vi "AOTF-Trigger_1.vi"(0 "Channel":string, 1 "Pulse length":i16[](array[numeric]), 2 "Sync trigger ratio":i32, 3 "error in (no error)":errorcluster caption="Fehler (Eingang, kein Fehler)", 4 "Triggered":bool, 5 "lp":dbl, 6 "ap":dbl) -> (7 "error out":errorcluster caption="Fehler (Ausgang)")   [LabVIEW 2009]
doc: "I. Description:\nThis example demonstrates how to generate a continuous digital pulse train from a Counter Output Channel started by an external digital trigger. The Frequency, Duty Cycle, and Idle State are all configurable. \n\nThis example shows how to configure the pulse in terms of Frequency/Duty Cycle, but can easily be modified to generate a pulse in terms of Time or Ticks.\n\nII. Instructions for Running:\n1. Select the Physical Channel which corresponds to the counter you want to output your signal to on the DAQ device.\n2. Enter the Frequency and Duty Cycle to define the pulse parameters. You can also change the Idle State to set the state the line will remain in after the generation is stopped. Additionally, you can set the Initial Delay (in seconds) which will delay the beginning of the pulse train from the start call; this is currently wired to 0.0 on the block diagram. \n3. Setup the Trigger Parameters. In this example the VI is expecting a Rising Edge Digital Trigger on PFI9. \n\nIII. Block Diagram Steps:\n1. Create a Counter Output channel to produce a Pulse in terms of Frequency. If the Idle State of the pulse is set to low the first transition of the generated signal is from low to high.\n2. Use the DAQmx Trigger VI to configure a trigger to start on a digital edge.\n2. Use the DAQmx Timing VI (Implicit) to configure the duration of the pulse generation.\n3. Call the Start VI to arm the counter and begin the pulse train generation.\n4. Loop continuously until the user presses the Stop button. Check for errors every 100 ms using the Is Task Done? VI\n5. Call the Clear Task VI to clear the Task.\n\nIV. I/O Connections Overview:\nThe counter will output the pulse train on the output terminal of the counter specified in the Physical Channel I/O control. \n\nIn this example the output will be sent to the default output terminal on ctr0.\n\nFor more information on the default counter input and output terminals for your device, open the NI-DAQmx Help, and refer to Counter Signal Connections found under the Device Considerations book in the table of contents."
uses:
  <vilib>/DAQmx/configure/timing.llb/DAQmx Timing (Implicit).vi
  <vilib>/Utility/error.llb/DialogType.ctl
  <vilib>/DAQmx/configure/trigger.llb/DAQmx Start Trigger (Digital Edge).vi
  <vilib>/DAQmx/write.llb/DAQmx Write (Digital Bool 1Line 1Point).vi
  <vilib>/DAQmx/read.llb/DAQmx Read (Digital Bool 1Line 1Point).vi
  <vilib>/DAQmx/create/channels.llb/DAQmx Create Channel (DI-Digital Input).vi
  <vilib>/DAQmx/create/channels.llb/DAQmx Create Channel (DO-Digital Output).vi
  <vilib>/DAQmx/create/channels.llb/DAQmx Create Channel (CO-Pulse Generation-Ticks).vi
  <vilib>/DAQmx/create/channels.llb/DAQmx Create Channel (CO-Pulse Generation-Frequency).vi
  <vilib>/DAQmx/create/channels.llb/DAQmx Create Channel (CO-Pulse Generation-Time).vi
panel:
  out "Delay":dbl[](array[numeric])
  out "Duty cycle":dbl[](array[numeric])
  # "Channel Parameters"
  # "Trigger Parameters"
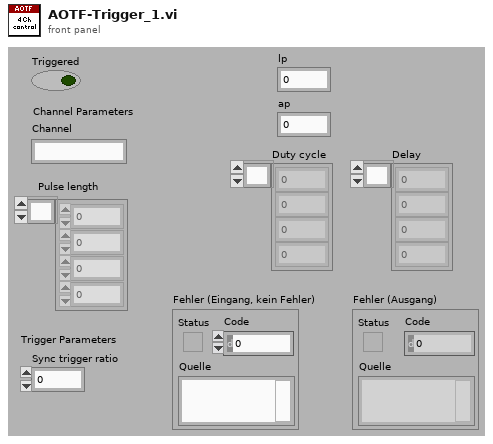
[diagram p1: front panel]
types:
  T1 = typedef "DialogType.ctl" = u16
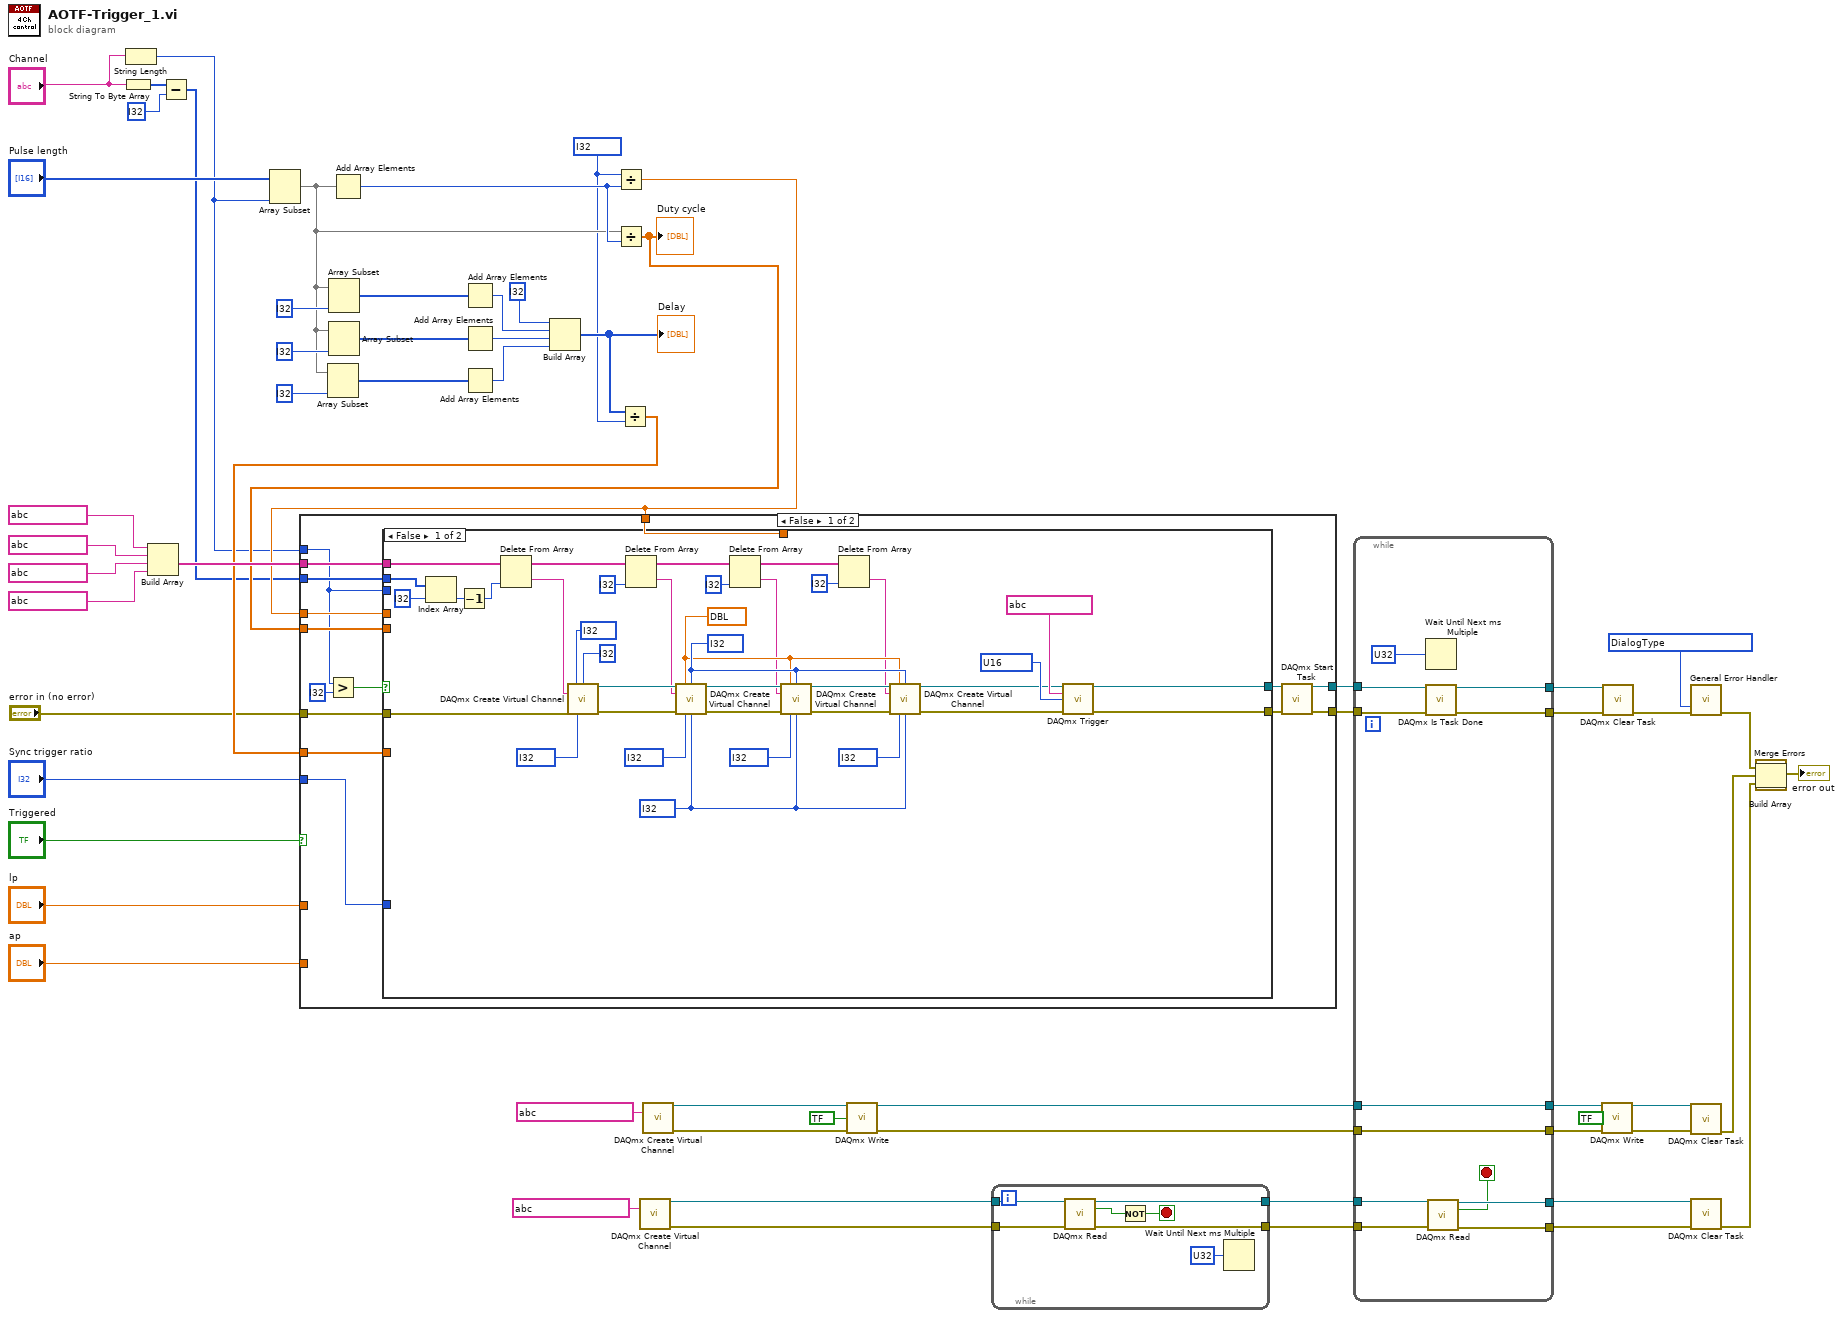
[diagram p0: block diagram]
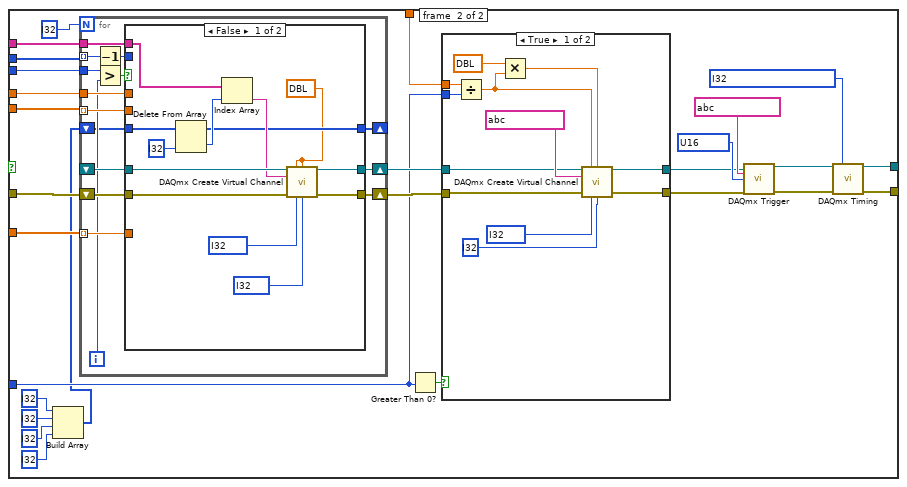
[diagram p2: hidden frame]
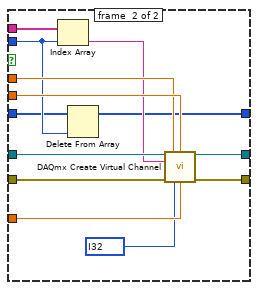
[diagram p4: hidden frame]
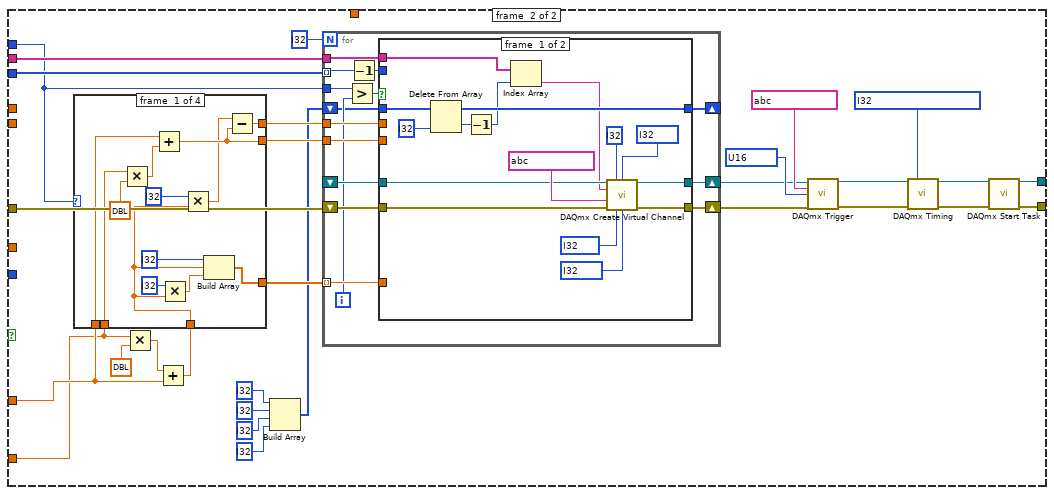
[diagram p5: hidden frame]
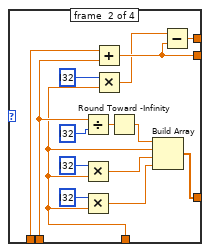
[diagram p6: hidden frame]
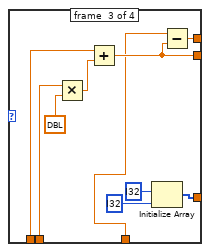
[diagram p7: hidden frame]
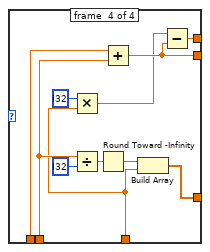
[diagram p8: hidden frame]
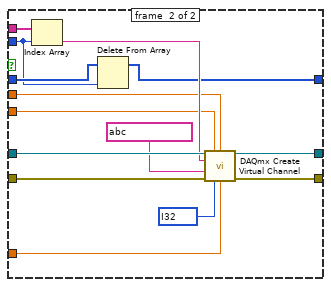
[diagram p9: hidden frame]
diagram:
  w39 = T1 ? items=["no dialog", "OK message", "continue or stop message", "OK message + warnings", "continue/stop + warnings"] ("type of dialog (OK msg:1)")
  w41 = i32 ?
  n1 = String To Byte Array(string="Channel") -> (unsigned byte array=w61:u8[])
  n2 = String Length(string="Channel") -> (length=w3:i32)
  n3 = Build Array(tag ? ("Counter 2"), tag ? ("Counter 2"), tag ? ("Counter 2"), tag ? ("Counter 2")) -> (w16:tag[])
  n4 = Subtract(x=w61, y=i32 ?) -> (x-y=w2:i32[])
  n5 = Array Subset(array="Pulse length", length=w3) -> (w43:i16[])  [unwired: 1 in]
  n6 = Array Subset(array=w43, length=i32 ?) -> (w53:i16[])  [unwired: 1 in]
  n7 = Array Subset(array=w43, length=i32 ?) -> (w52:i16[])  [unwired: 1 in]
  n8 = Array Subset(array=w43, length=i32 ?) -> (w54:i16[])  [unwired: 1 in]
  n9 = Add Array Elements(numeric array=w43) -> (sum=w44:i16)
  n10 = Add Array Elements(numeric array=w52) -> (sum=w49:i16)
  n11 = Add Array Elements(numeric array=w54) -> (sum=w51:i16)
  n12 = Add Array Elements(numeric array=w53) -> (sum=w50:i16)
  n13 = Build Array(i32 ?, w49, w51, w50) -> (w42:i32[])
  "Delay" <- w42
  n14 = Divide(x=w41, y=w44) -> (x/y=w12:dbl)
  n15 = Divide(x=w43, y=w44) -> (x/y=w14:dbl[])
  "Duty cycle" <- w14
  n16 = Divide(x=w42, y=w41) -> (x/y=w15:dbl[])
  n17 = case shown="False" "Triggered" {
    tunnel: [w75 w225] -> w36
    tunnel: [w74 w224] -> w35
    tunnel: w16 -> [w72 w206]
    tunnel: w2 -> [w68 w216]
    tunnel: w15 -> [w71 _]
    tunnel: w14 -> [w69 _]
    tunnel: w12 -> [w70 _]
    tunnel: w3 -> [w64 w202]
    tunnel: "Sync trigger ratio" -> [w73 _]
    tunnel: w12 -> [w67 _]
    tunnel: "error in (no error)" -> [w66 w215]
    tunnel: "ap" -> [_ w209]
    tunnel: "lp" -> [_ w210]
    frame #0 {
      n18 = Greater?(x=w64, y=i32 ?) -> (0:w65:bool)
      n19 = case shown="False" w65 {
        tunnel: [w109 w141] -> w77
        tunnel: [w110 w140] -> w76
        tunnel: w73 -> [_ w131]
        tunnel: w72 -> [w112 w128]
        tunnel: w71 -> [_ w127]
        tunnel: w70 -> [_ w126]
        tunnel: w69 -> [_ w125]
        tunnel: w68 -> [w104 w124]
        tunnel: w64 -> [_ w117]
        tunnel: w67 -> [_ w123]
        tunnel: w66 -> [w111 w122]
        frame #0 {
          w89 = i32 ?
          w98 = i32 ? items=["High", "Low"] ("Idle State 2")
          w99 = i32 ? items=["High", "Low"] ("Idle State 2")
          w100 = i32 ? items=["High", "Low"] ("Idle State 2")
          w88 = i32 ?
          w87 = dbl ?
          w105 = i32 ? items=["High", "Low"] ("Idle State 2")
          w113 = u16 ? items=["Falling", "Rising"]
          n20 = Index Array(array=w104, index=i32 ?) -> (element=w102:i32)
          n21 = Decrement(x=w102) -> (x-1=w101:i32)
          n22 = Delete From Array(array=w112, index=w101) -> (deleted portion=w108:tag, array with subset deleted=w86:tag[])  [unwired: 1 in]
          n23 = call-poly <vilib>:"DAQmx Create Virtual Channel.vi"("high time"=i32 ?, "low time"=i32 ?, "counter"=w108, "error in"=w111, "idle state"=w105) -> ("task out"=w90:refnum<k21>, "error out"=w97:errorcluster)  [unwired: 9 in]
          n24 = Delete From Array(array=w86, index=i32 ?) -> (deleted portion=w82:tag, array with subset deleted=w85:tag[])  [unwired: 1 in]
          n25 = call-poly <vilib>:"DAQmx Create Virtual Channel.vi"("task in"=w90, "high time"=w87, "low time"=w88, "counter"=w82, "error in"=w97, "idle state"=w100, "initial delay"=w89) -> ("task out"=w91:refnum<k21>, "error out"=w96:errorcluster)  [unwired: 7 in]
          n26 = Delete From Array(array=w85, index=i32 ?) -> (deleted portion=w81:tag, array with subset deleted=w84:tag[])  [unwired: 1 in]
          n27 = call-poly <vilib>:"DAQmx Create Virtual Channel.vi"("task in"=w91, "high time"=w87, "low time"=w88, "counter"=w81, "error in"=w96, "idle state"=w99, "initial delay"=w89) -> ("task out"=w92:refnum<k21>, "error out"=w95:errorcluster)  [unwired: 7 in]
          n28 = Delete From Array(array=w84, index=i32 ?) -> (deleted portion=w83:tag)  [unwired: 1 in, 1 out]
          n29 = call-poly <vilib>:"DAQmx Create Virtual Channel.vi"("task in"=w92, "high time"=w87, "low time"=w88, "counter"=w83, "error in"=w95, "idle state"=w98, "initial delay"=w89) -> ("task out"=w93:refnum<k21>, "error out"=w94:errorcluster)  [unwired: 7 in]
          n30 = call-poly <vilib>:"DAQmx Trigger.vi"("task/channels in"=w93, "source"=tag ? ("Trigger Source"), "edge"=w113, "error in"=w94) -> ("task out"=w110:refnum<k21>, "error out"=w109:errorcluster)  [unwired: 10 in]
        }
        frame #1 {
          w137 = u16 ? items=["Falling", "Rising"]
          w139 = i32 ? items=["Finite Samples", "Continuous Samples"] ("sample mode")
          n31 = Build Array(i32 ?, i32 ?, i32 ?, i32 ?) -> (w115:i32[])
          n32 = for {
            N: i32 ? -> [_]
            shift-right: [w170] -> w133
            shift-left: w122 -> [w169]
            shift-right: [w168] -> w132
            shift-left: _ -> [w167]
            tunnel: w125 -> [w166] mode=indexing
            tunnel: w126 -> [w165]
            tunnel: w127 -> [w164] mode=indexing
            tunnel: w128 -> [w163]
            tunnel: w124 -> [w162] mode=indexing
            tunnel: w117 -> [w159]
            shift-right: [w156] -> _
            shift-left: w115 -> [w157]
            i -> [w160]
            n33 = Decrement(x=w162) -> (x-1=w158:i32)
            n34 = Greater?(x=w159, y=w160) -> (0:w161:bool)
            n35 = case shown="False" w161 {
              tunnel: [w182 w196] -> w170
              tunnel: w169 -> [w181 w195]
              tunnel: [w179 w194] -> w168
              tunnel: w167 -> [w180 w193]
              tunnel: w166 -> [_ w192]
              tunnel: w165 -> [_ w191]
              tunnel: w164 -> [_ w190]
              tunnel: w163 -> [w175 w188]
              tunnel: w158 -> [_ w186]
              tunnel: w157 -> [w177 w185]
              tunnel: [w173 w184] -> w156
              frame #0 {
                w171 = dbl ?
                w183 = i32 ? items=["High", "Low"] ("Idle State 2")
                n36 = Delete From Array(array=w177, index=i32 ?) -> (deleted portion=w176:i32, array with subset deleted=w173:i32[])  [unwired: 1 in]
                n37 = Index Array(array=w175, index=w176) -> (element=w174:tag)
                n38 = call-poly <vilib>:"DAQmx Create Virtual Channel.vi"("task in"=w180, "frequency"=w171, "duty cycle"=w171, "counter"=w174, "error in"=w181, "idle state"=w183, "initial delay"=i32 ?) -> ("task out"=w179:refnum<k21>, "error out"=w182:errorcluster)  [unwired: 7 in]
              }
              frame #1 {
                w187 = i32 ? items=["High", "Low"] ("Idle State 2")
                n39 = Index Array(array=w188, index=w186) -> (element=w189:tag)
                n40 = Delete From Array(array=w185, index=w186) -> (array with subset deleted=w184:i32[])  [unwired: 1 in, 1 out]
                n41 = call-poly <vilib>:"DAQmx Create Virtual Channel.vi"("task in"=w193, "frequency"=w191, "duty cycle"=w192, "counter"=w189, "error in"=w195, "idle state"=w187, "initial delay"=w190) -> ("task out"=w194:refnum<k21>, "error out"=w196:errorcluster)  [unwired: 7 in]
              }
            }
          }
          n42 = Greater Than 0?(x=w131) -> (x > 0?=w134:bool)
          n43 = case shown="True" w134 {
            tunnel: [w152 w155] -> w129
            tunnel: [w149 w154] -> w130
            tunnel: w123 -> [w148 _]
            tunnel: w131 -> [w147 _]
            tunnel: w133 -> [w143 w154]
            tunnel: w132 -> [w142 w155]
            frame #0 {
              w150 = i32 ? items=["High", "Low"] ("Idle State 2")
              n44 = Divide(x=w148, y=w147) -> (x/y=w144:dbl)
              n45 = Multiply(x=dbl ?, y=w144) -> (x*y=w146:dbl)
              n46 = call-poly <vilib>:"DAQmx Create Virtual Channel.vi"("task in"=w142, "frequency"=w144, "duty cycle"=w146, "counter"=tag ? ("Counter 2"), "error in"=w143, "idle state"=w150, "initial delay"=i32 ?) -> ("task out"=w152:refnum<k21>, "error out"=w149:errorcluster)  [unwired: 7 in]
            }
            frame #1 {
            }
          }
          n47 = call-poly <vilib>:"DAQmx Trigger.vi"("task/channels in"=w129, "source"=tag ? ("Trigger Source"), "edge"=w137, "error in"=w130) -> ("task out"=w135:refnum<k21>, "error out"=w136:errorcluster)  [unwired: 10 in]
          n48 = call-poly <vilib>:"DAQmx Timing.vi"("task/channels in"=w135, "sample mode"=w139, "error in"=w136) -> ("task out"=w140:refnum<k21>, "error out"=w141:errorcluster)  [unwired: 11 in]
        }
      }
      n49 = call <vilib>:"DAQmx Start Task.vi"("task/channels in"=w76, "error in"=w77) -> ("task out"=w74:refnum<k21>, "error out"=w75:errorcluster)  [unwired: 12 in]
    }
    frame #1 {
      w221 = u16 ? items=["Falling", "Rising"]
      w223 = i32 ? items=["Finite Samples", "Continuous Samples"] ("sample mode")
      n50 = Multiply(x=w209, y=dbl ?) -> (x*y=w211:dbl)
      n51 = Add(x=w211, y=w210) -> (x+y=w208:dbl)
      n52 = case shown="1, Default" w202 {
        tunnel: w209 -> [w234 w249 w262 w269]
        tunnel: [w230 w245 w255 w268] -> w207
        tunnel: [w235 w248 w258 w271] -> w214
        tunnel: [w236 w251 w259 w272] -> w213
        tunnel: w210 -> [w233 w250 w263 w270]
        tunnel: w208 -> [w227 w239 w254 w265]
        frame #0 {
          n53 = Multiply(x=w234, y=dbl ?) -> (x*y=w237:dbl)
          n54 = Add(x=w233, y=w237) -> (x+y=w235:dbl)
          n55 = Multiply(x=i32 ?, y=w227) -> (x*y=w228:dbl)
          n56 = Multiply(x=i32 ?, y=w227) -> (x*y=w231:dbl)
          n57 = Build Array(i32 ?, w227, w228) -> (w230:dbl[])
          n58 = Subtract(x=w231, y=w235) -> (x-y=w236:dbl)
        }
        frame #1 {
          n59 = Divide(x=w249, y=i32 ?) -> (x/y=w252:dbl)
          n60 = Multiply(x=i32 ?, y=w239) -> (x*y=w242:dbl)
          n61 = Multiply(x=i32 ?, y=w239) -> (x*y=w241:dbl)
          n62 = Add(x=w250, y=w249) -> (x+y=w248:dbl)
          n63 = Multiply(x=i32 ?, y=w239) -> (x*y=w246:dbl)
          n64 = Round Toward -Infinity(1:w252) -> (0:w244:dbl)
          n65 = Build Array(w244, w239, w242, w241) -> (w245:dbl[])
          n66 = Subtract(x=w246, y=w248) -> (x-y=w251:dbl)
        }
        frame #2 {
          n67 = Multiply(x=w262, y=dbl ?) -> (x*y=w260:dbl)
          n68 = Add(x=w263, y=w260) -> (x+y=w258:dbl)
          n69 = Initialize Array(i32 ?, i32 ?) -> (w255:i32[])
          n70 = Subtract(x=w254, y=w258) -> (x-y=w259:dbl)
        }
        frame #3 {
          n71 = Multiply(x=i32 ?, y=w265) -> (x*y=w266:dbl)
          n72 = Divide(x=w269, y=i32 ?) -> (x/y=w273:dbl)
          n73 = Round Toward -Infinity(1:w273) -> (0:w267:dbl)
          n74 = Add(x=w270, y=w269) -> (x+y=w271:dbl)
          n75 = Build Array(w267, w265) -> (w268:dbl[])
          n76 = Subtract(x=w266, y=w271) -> (x-y=w272:dbl)
        }
      }
      n77 = Build Array(i32 ?, i32 ?, i32 ?, i32 ?) -> (w197:i32[])
      n78 = for {
        N: i32 ? -> [_]
        shift-right: [w289] -> w204
        shift-left: w215 -> [w288]
        shift-right: [w287] -> w205
        shift-left: _ -> [w286]
        tunnel: w206 -> [w284]
        tunnel: w216 -> [w277] mode=indexing
        tunnel: w207 -> [w283] mode=indexing
        tunnel: w214 -> [w282]
        tunnel: w213 -> [w281]
        tunnel: w202 -> [w278]
        shift-right: [w275] -> _
        shift-left: w197 -> [w276]
        i -> [w279]
        n79 = Greater?(x=w278, y=w279) -> (0:w280:bool)
        n80 = Decrement(x=w277) -> (x-1=w285:i32)
        n81 = case shown="True" w280 {
          tunnel: [w302 w319] -> w289
          tunnel: w288 -> [w303 w318]
          tunnel: [w300 w317] -> w287
          tunnel: w286 -> [w301 w316]
          tunnel: w285 -> [_ w307]
          tunnel: w284 -> [w296 w312]
          tunnel: w283 -> [_ w311]
          tunnel: w282 -> [_ w310]
          tunnel: w281 -> [_ w309]
          tunnel: w276 -> [w299 w308]
          tunnel: [w297 w306] -> w275
          frame #0 {
            w304 = i32 ? items=["High", "Low"] ("Idle State 2")
            n82 = Delete From Array(array=w299, index=i32 ?) -> (deleted portion=w295:i32, array with subset deleted=w297:i32[])  [unwired: 1 in]
            n83 = Decrement(x=w295) -> (x-1=w294:i32)
            n84 = Index Array(array=w296, index=w294) -> (element=w293:tag)
            n85 = call-poly <vilib>:"DAQmx Create Virtual Channel.vi"("task in"=w301, "high ticks"=i32 ?, "low ticks"=i32 ?, "counter"=w293, "source of ticks"=tag ? ("Trigger Source"), "error in"=w303, "idle state"=w304, "initial delay"=i32 ?) -> ("task out"=w300:refnum<k21>, "error out"=w302:errorcluster)  [unwired: 6 in]
          }
          frame #1 {
            w313 = i32 ? items=["High", "Low"] ("Idle State 2")
            n86 = Index Array(array=w312, index=w307) -> (element=w315:tag)
            n87 = Delete From Array(array=w308, index=w307) -> (array with subset deleted=w306:i32[])  [unwired: 1 in, 1 out]
            n88 = call-poly <vilib>:"DAQmx Create Virtual Channel.vi"("task in"=w316, "high ticks"=w310, "low ticks"=w309, "counter"=w315, "source of ticks"=tag ? ("Trigger Source"), "error in"=w318, "idle state"=w313, "initial delay"=w311) -> ("task out"=w317:refnum<k21>, "error out"=w319:errorcluster)  [unwired: 6 in]
          }
        }
      }
      n89 = call-poly <vilib>:"DAQmx Trigger.vi"("task/channels in"=w205, "source"=tag ? ("Trigger Source"), "edge"=w221, "error in"=w204) -> ("task out"=w218:refnum<k21>, "error out"=w217:errorcluster)  [unwired: 10 in]
      n90 = call-poly <vilib>:"DAQmx Timing.vi"("task/channels in"=w218, "sample mode"=w223, "error in"=w217) -> ("task out"=w220:refnum<k21>, "error out"=w219:errorcluster)  [unwired: 11 in]
      n91 = call <vilib>:"DAQmx Start Task.vi"("task/channels in"=w220, "error in"=w219) -> ("task out"=w224:refnum<k21>, "error out"=w225:errorcluster)  [unwired: 12 in]
    }
  }
  n92 = call-poly <vilib>:"DAQmx Create Virtual Channel.vi"("lines"=tag ? ("Counter 2")) -> ("task out"=w22:refnum<k21>, "error out"=w21:errorcluster)  [unwired: 13 in]
  n93 = call-poly <vilib>:"DAQmx Create Virtual Channel.vi"("lines"=tag ? ("Counter 2")) -> ("task out"=w17:refnum<k21>, "error out"=w18:errorcluster)  [unwired: 13 in]
  n94 = call-poly <vilib>:"DAQmx Write.vi"("task/channels in"=w17, "data"=bool ?, "error in"=w18) -> ("task out"=w25:refnum<k21>, "error out"=w26:errorcluster)  [unwired: 10 in, 1 out]
  n95 = while {
    tunnel: w22 -> [w326]
    tunnel: w21 -> [w325]
    tunnel: [w324] -> w20
    tunnel: [w323] -> w19
    stop <- w320 stop-if-true
    n96 = call-poly <vilib>:"DAQmx Read.vi"("task/channels in"=w326, "error in"=w325) -> ("task out"=w323:refnum<k21>, "data"=w321:bool, "error out"=w324:errorcluster)  [unwired: 11 in]
    n97 = Not(x=w321) -> (.not. x?=w320:bool)
    n98 = Wait Until Next ms Multiple(millisecond multiple=u32 ?) -> ()  [unwired: 1 out]
  }
  n99 = while {
    tunnel: w36 -> [w337]
    tunnel: w35 -> [w338]
    tunnel: [w336] -> w37
    tunnel: [w335] -> w38
    tunnel: w19 -> [w331]
    tunnel: w20 -> [w330]
    tunnel: [w327] -> w30
    tunnel: [w328] -> w29
    tunnel: w25 -> [w328]
    tunnel: w26 -> [w327]
    tunnel: [w333] -> w23
    tunnel: [w332] -> w24
    stop <- w329 stop-if-true
    n100 = Wait Until Next ms Multiple(millisecond multiple=u32 ?) -> ()  [unwired: 1 out]
    n101 = call <vilib>:"DAQmx Is Task Done.vi"("task/channels in"=w338, "error in"=w337) -> ("task out"=w336:refnum<k21>, "error out"=w335:errorcluster)  [unwired: 11 in, 1 out]
    n102 = call-poly <vilib>:"DAQmx Read.vi"("task/channels in"=w331, "error in"=w330) -> ("task out"=w332:refnum<k21>, "data"=w329:bool, "error out"=w333:errorcluster)  [unwired: 11 in]
  }
  n103 = call-poly <vilib>:"DAQmx Write.vi"("task/channels in"=w29, "data"=bool ?, "error in"=w30) -> ("task out"=w32:refnum<k21>, "error out"=w31:errorcluster)  [unwired: 10 in, 1 out]
  n104 = call <vilib>:"DAQmx Clear Task.vi"("task in"=w37, "error in"=w38) -> ("error out"=w62:errorcluster)  [unwired: 13 in]
  n105 = call <vilib>:"General Error Handler.vi"("type of dialog (OK msg:1)"=w39, "error in (no error)"=w62) -> ("error out"=w11:errorcluster)  [unwired: 9 in, 4 out]
  n106 = call <vilib>:"DAQmx Clear Task.vi"("task in"=w32, "error in"=w31) -> ("error out"=w10:errorcluster)  [unwired: 13 in]
  n107 = call <vilib>:"DAQmx Clear Task.vi"("task in"=w24, "error in"=w23) -> ("error out"=w9:errorcluster)  [unwired: 13 in]
  n108 = Build Array(w11, w10, w9) -> (w1:errorcluster[])
  n109 = call <vilib>:"Merge Errors.vi"("error array in"=w1) -> ("error out"=→"error out":errorcluster)  [unwired: 6 in]
